vi "Init Queues Command Based Example.vi"(8 "error in (no error)":errorcluster) -> (0 "error out":errorcluster, 3 "Queue Refs":T1)   [LabVIEW 2020]
doc: "Copyright 2015, 2016, 2017 National Instruments Corporation\n\nLicensed under the Apache License, Version 2.0 (the \"License\"); you may not use this file except in compliance with the License.\n\n You may obtain a copy of the License at\n\n http://www.apache.org/licenses/LICENSE-2.0\n\nUnless required by applicable law or agreed to in writing, software distributed under the License is distributed on an \"AS IS\" BASIS, WITHOUT WARRANTIES OR CONDITIONS OF ANY KIND, either express or implied.\n\nSee the License for the specific language governing permissions and limitations under the License."
uses:
  Command Based Example Queue Refs.ctl
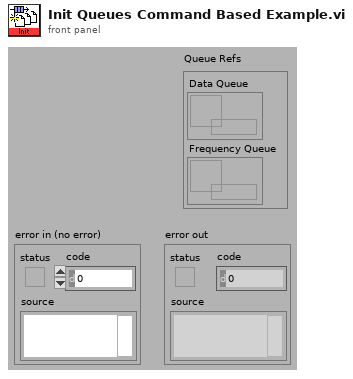
[diagram p1: front panel]
types:
  T1 = typedef "Command Based Example Queue Refs.ctl" = cluster{"Data Queue":refnum<queue>, "Frequency Queue":refnum<queue>}
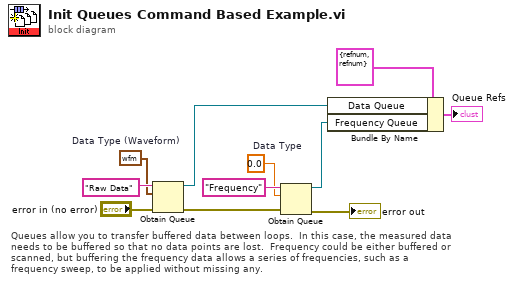
[diagram p0: block diagram]
diagram:
  w6 = waveform(dbl) {"t0"=timestamp(0 s since 1904-01-01), "dt"=1.0, "Y"=[]}  # Data Type (Waveform)
  w5 = 0.0  # Data Type
  # "Queues allow you to transfer buffered data between loops.  In this case, the measured data needs to be buffered so that no data points are lost.  Frequency could be either buffered or scanned, but buffering the frequency data allows a series of frequencies, such as a frequency sweep, to be applied without missing any."
  n1 = Obtain Queue(name (unnamed)="Raw Data", element data type=w6, error in (no error)="error in (no error)") -> (queue out=w3:refnum<queue>, error out=w8:errorcluster)  [unwired: 2 in, 1 out]
  n2 = Obtain Queue(name (unnamed)="Frequency", element data type=w5, error in (no error)=w8) -> (queue out=w2:refnum<queue>, error out=→"error out":errorcluster)  [unwired: 2 in, 1 out]
  n3 = Bundle By Name(cluster=T1 {"Data Queue"=refnum, "Frequency Queue"=refnum} ("Queue Refs"), "Data Queue"=w3, "Frequency Queue"=w2) -> (→"Queue Refs":T1)
